vi "panic.vi"(2 "inputSpeed":cluster{"left":dbl, "right":dbl}={"left"=1.0, "right"=-1.0}, 3 "panic":bool) -> (0 "output speed":cluster{"left":dbl, "right":dbl}={"left"=1.0, "right"=-1.0})   [LabVIEW 2016]
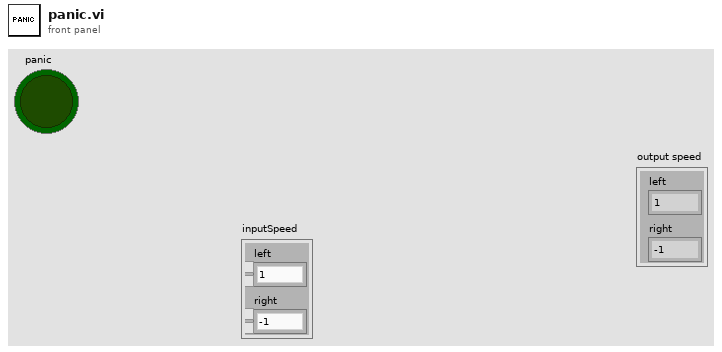
[diagram p1: front panel]
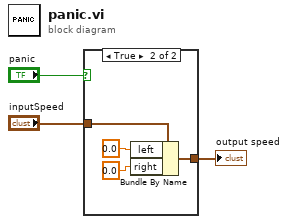
[diagram p0: block diagram]
diagram:
  n1 = case shown="True" "panic" {
    tunnel: [w4 w7] -> w3
    tunnel: "inputSpeed" -> [w4 w8]
    frame False {
    }
    frame True {
      n2 = Bundle By Name(cluster=w8, "left"=0.0, "right"=0.0) -> (w7:cluster{"left":dbl, "right":dbl})
    }
  }
  "output speed" <- w3
